vi "NADC Freq Channels.vi"(7 "Channel Number (1)":i16=1, 8 "error in (no error)":errorcluster {"code" format="%.0x"}, 9 "Channel Band (T:BASE)":bool=TRUE, 10 "Freq Channels (F:OFF)":bool, 11 "VISA Resource Name":refnum<visa-resource-name>) -> (0 "error out":errorcluster {"code" format="%.0x"}, 3 "VISA Resource Name Out":refnum<visa-resource-name>)   [LabVIEW 2012, in "Agilent ESG Series.lvlib"]
doc: "This VI is used to configure the \"Freq Channels\" parameters."
uses:
  <instrlib>/Agilent ESG Series/Agilent ESG Series.lvlib
panel:
  # "ON"
  # "OFF"
  # "BASE"
  # "MOBILE"
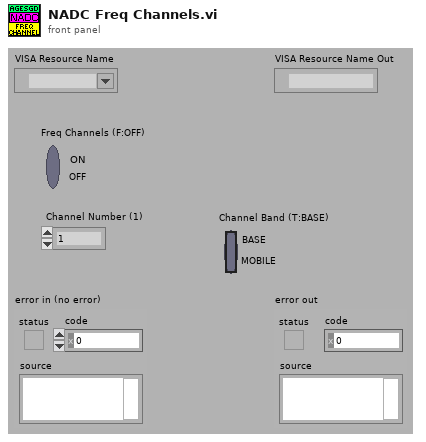
[diagram p1: front panel]
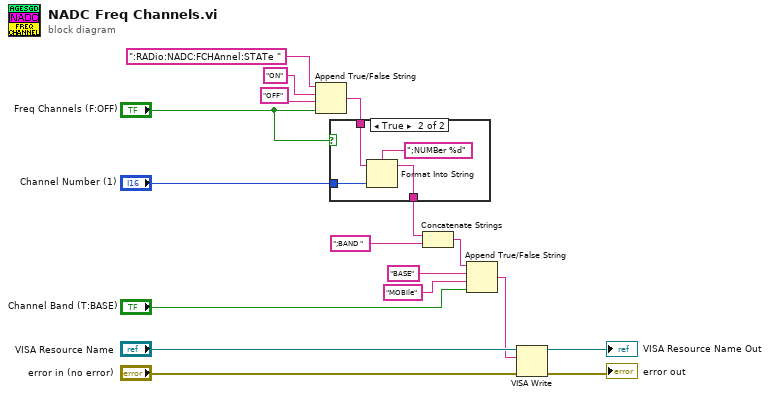
[diagram p0: block diagram]
diagram:
  n1 = Append True/False String(1:"Freq Channels (F:OFF)", 2:"OFF" ("false string"), 3:"ON" ("true string"), 4:":RADio:NADC:FCHAnnel:STATe ") -> (0:w11:string)
  n2 = case shown="True" "Freq Channels (F:OFF)" {
    tunnel: [w18 w21] -> w6
    tunnel: w11 -> [w18 w20]
    tunnel: "Channel Number (1)" -> [_ w19]
    frame False {
    }
    frame True {
      n3 = Format Into String(format string=";NUMBer %d", initial string=w20, w19) -> (resulting string=w21:string)  [unwired: 1 in, 1 out]
    }
  }
  n4 = Concatenate Strings(w6, ";BAND ") -> (w7:string)
  n5 = Append True/False String(1:"Channel Band (T:BASE)", 2:"MOBile" ("false string"), 3:"BASE" ("true string"), 4:w7) -> (0:w4:string)
  n6 = VISA Write(VISA resource name="VISA Resource Name", write buffer=w4, error in (no error)="error in (no error)") -> (VISA resource name out=→"VISA Resource Name Out":refnum<visa-resource-name>, error out=→"error out":errorcluster)  [unwired: 1 out]
